vi "DriveNetwork_ReadSlow.vi"(8 "error in (no error)":errorcluster) -> (0 "error out":errorcluster)   [LabVIEW 2023]
doc: "Network for Drive\n\nInputs:\n -- Error in -- Error cluster -- propagated error input\n\nOutputs:\n -- Error out -- Error cluster -- progated error output"
uses:
  DriveGlobal.vi
  <vilib>/Rock Robotics/Network Tables/NT Read Boolean.vi
  <vilib>/Rock Robotics/Network Tables/NT Write Boolean.vi
  <vilib>/Rock Robotics/Network Tables/NT Read Number.vi
  <vilib>/Rock Robotics/Network Tables/NT Write Number.vi
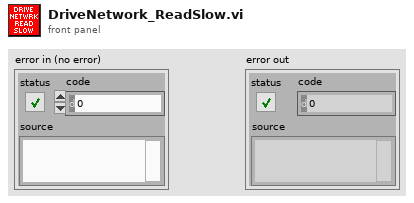
[diagram p1: front panel]
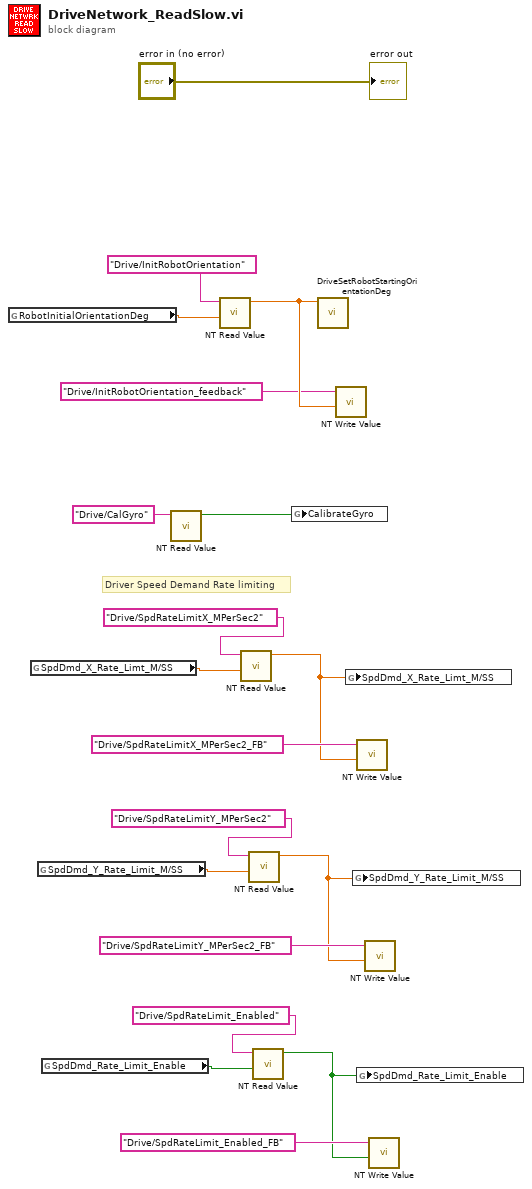
[diagram p0: block diagram]
diagram:
  # "Driver Speed Demand Rate limiting"
  n1 = global read "DriveGlobal.vi" "RobotInitialOrientationDeg"() -> (w13:dbl)
  n2 = global read "DriveGlobal.vi" "SpdDmd_X_Rate_Limt_M/SS"() -> (w11:dbl)
  n3 = global read "DriveGlobal.vi" "SpdDmd_Y_Rate_Limit_M/SS"() -> (w7:dbl)
  n4 = global read "DriveGlobal.vi" "SpdDmd_Rate_Limit_Enable"() -> (w3:bool)
  n5 = call-poly <vilib>:"NT Read Value.vi"("name"="Drive/CalGyro") -> ("value"=w17:bool)  [unwired: 8 in, 2 out]
  n6 = call-poly <vilib>:"NT Read Value.vi"("default value"=w13, "name"="Drive/InitRobotOrientation") -> ("value"=w15:dbl)  [unwired: 7 in, 2 out]
  n7 = call-poly <vilib>:"NT Read Value.vi"("default value"=w11, "name"="Drive/SpdRateLimitX_MPerSec2") -> ("value"=w9:dbl)  [unwired: 7 in, 2 out]
  n8 = call-poly <vilib>:"NT Read Value.vi"("default value"=w7, "name"="Drive/SpdRateLimitY_MPerSec2") -> ("value"=w5:dbl)  [unwired: 7 in, 2 out]
  n9 = call-poly <vilib>:"NT Read Value.vi"("default value"=w3, "name"="Drive/SpdRateLimit_Enabled") -> ("value"=w1:bool)  [unwired: 7 in, 2 out]
  n10 = global write "DriveGlobal.vi" "CalibrateGyro"(w17) -> ()
  n11 = call "DriveSetRobotStartingOrientationDeg.vi"("GyroIntDirection"=w15) -> ()  [unwired: 11 in]
  n12 = call-poly <vilib>:"NT Write Value.vi"("value"=w15, "name"="Drive/InitRobotOrientation_feedback") -> ()  [unwired: 9 in, 1 out]
  n13 = global write "DriveGlobal.vi" "SpdDmd_X_Rate_Limt_M/SS"(w9) -> ()
  n14 = global write "DriveGlobal.vi" "SpdDmd_Y_Rate_Limit_M/SS"(w5) -> ()
  n15 = call-poly <vilib>:"NT Write Value.vi"("value"=w9, "name"="Drive/SpdRateLimitX_MPerSec2_FB") -> ()  [unwired: 9 in, 1 out]
  n16 = global write "DriveGlobal.vi" "SpdDmd_Rate_Limit_Enable"(w1) -> ()
  n17 = call-poly <vilib>:"NT Write Value.vi"("value"=w5, "name"="Drive/SpdRateLimitY_MPerSec2_FB") -> ()  [unwired: 9 in, 1 out]
  n18 = call-poly <vilib>:"NT Write Value.vi"("value"=w1, "name"="Drive/SpdRateLimit_Enabled_FB") -> ()  [unwired: 9 in, 1 out]
  "error out" <- "error in (no error)"
